vi "Save As CSV.vi"(8 "error in (no error)":errorcluster caption="错误输入（无错误）", 10 "dup path":path, 11 "从板个数":i32) -> (0 "error out":errorcluster caption="错误输出")   [LabVIEW 2013]
uses:
  <vilib>/Utility/file.llb/Write To Spreadsheet File (string).vi
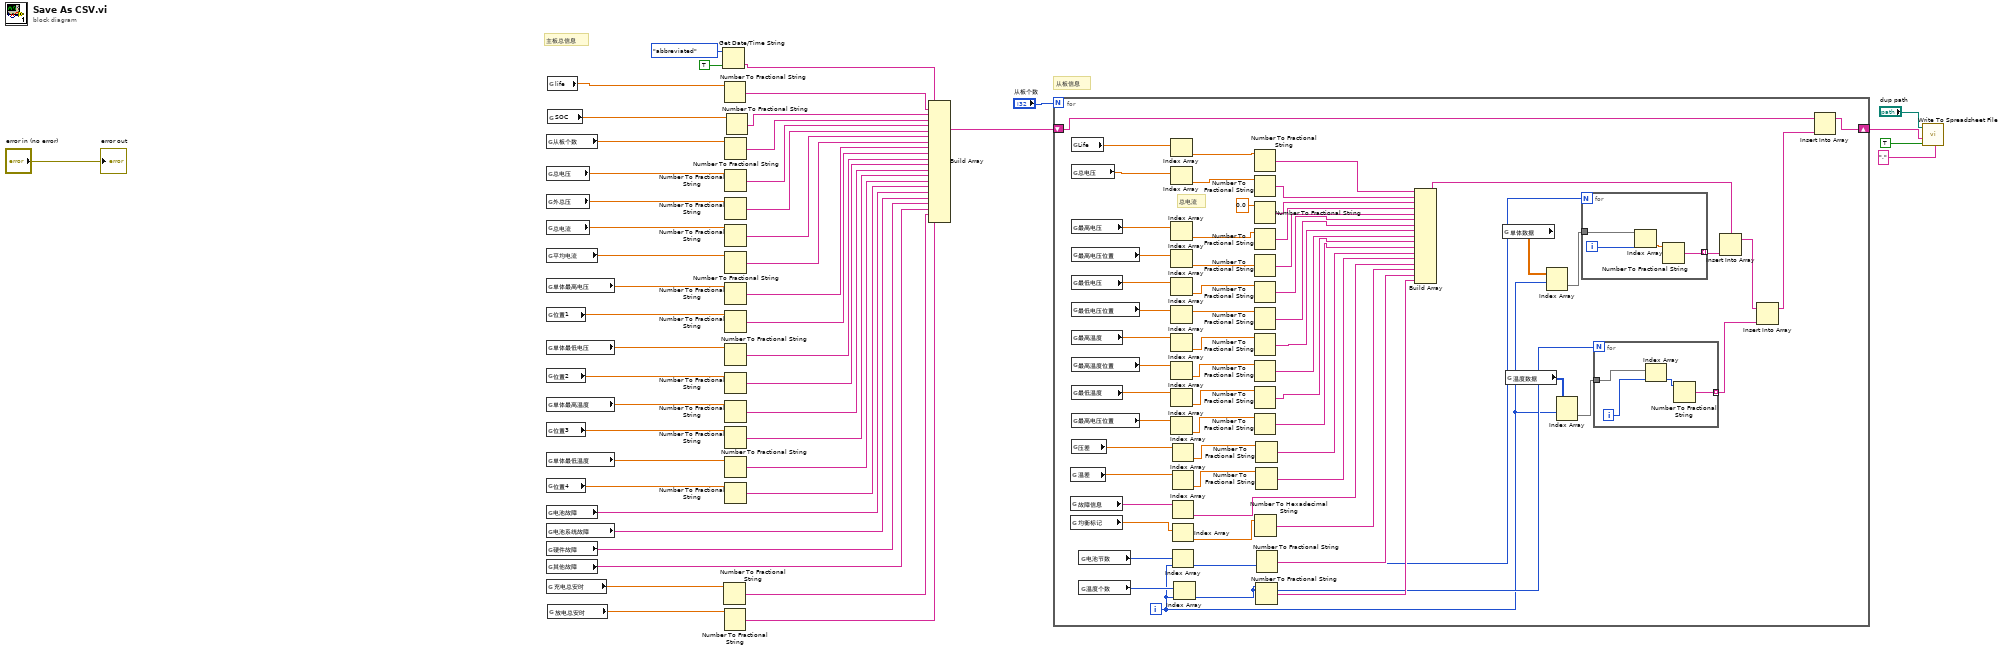
[diagram p0: block diagram]
diagram:
  # "从板信息"
  # "主板总信息"
  n1 = global read "电池信息全局变量.vi" "从板个数"() -> (w20:dbl)
  n2 = global read "EV05全局变量1.vi" "总电压"() -> (w27:dbl)
  n3 = global read "电池信息全局变量.vi" "外总压"() -> (w25:dbl)
  n4 = global read "EV05全局变量1.vi" "总电流"() -> (w26:dbl)
  n5 = global read "电池信息全局变量.vi" "平均电流"() -> (w24:dbl)
  n6 = global read "EV05全局变量1.vi" "单体最高电压"() -> (w17:dbl)
  n7 = global read "EV05全局变量1.vi" "位置1"() -> (w16:dbl)
  n8 = global read "EV05全局变量1.vi" "单体最低电压"() -> (w15:dbl)
  n9 = global read "EV05全局变量1.vi" "位置2"() -> (w14:dbl)
  n10 = global read "EV05全局变量1.vi" "单体最高温度"() -> (w13:dbl)
  n11 = global read "EV05全局变量1.vi" "位置3"() -> (w12:dbl)
  n12 = global read "EV05全局变量1.vi" "单体最低温度"() -> (w11:dbl)
  n13 = global read "EV05全局变量1.vi" "位置4"() -> (w10:dbl)
  n14 = global read "EV05全局变量1.vi" "电池故障"() -> (w9:string)
  n15 = global read "EV05全局变量1.vi" "电池系统故障"() -> (w8:string)
  n16 = global read "EV05全局变量1.vi" "硬件故障"() -> (w7:string)
  n17 = global read "EV05全局变量1.vi" "其他故障"() -> (w6:string)
  n18 = global read "电池信息全局变量.vi" "充电总安时"() -> (w4:dbl)
  n19 = global read "EV05全局变量1.vi" "life"() -> (w19:dbl)
  n20 = global read "EV05全局变量1.vi" "SOC"() -> (w18:dbl)
  n21 = global read "电池信息全局变量.vi" "放电总安时"() -> (w5:dbl)
  n22 = Get Date/Time String(date format (0)=enum16{"short", "long", "abbreviated"}."abbreviated" ("日期格式(0)"), want seconds? (F)=TRUE ("需要秒？(F)")) -> (time string=w46:string)  [unwired: 1 in, 1 out]
  n23 = Number To Fractional String(number=w4) -> (F-format string=w29:string)  [unwired: 3 in]
  n24 = Number To Fractional String(number=w19) -> (F-format string=w3:string)  [unwired: 3 in]
  n25 = Number To Fractional String(number=w5) -> (F-format string=w28:string)  [unwired: 3 in]
  n26 = Number To Fractional String(number=w20) -> (F-format string=w45:string)  [unwired: 3 in]
  n27 = Number To Fractional String(number=w27) -> (F-format string=w44:string)  [unwired: 3 in]
  n28 = Number To Fractional String(number=w25) -> (F-format string=w23:string)  [unwired: 3 in]
  n29 = Number To Fractional String(number=w26) -> (F-format string=w43:string)  [unwired: 3 in]
  n30 = Number To Fractional String(number=w24) -> (F-format string=w22:string)  [unwired: 3 in]
  n31 = Number To Fractional String(number=w17) -> (F-format string=w41:string)  [unwired: 3 in]
  n32 = Number To Fractional String(number=w16) -> (F-format string=w40:string)  [unwired: 3 in]
  n33 = Number To Fractional String(number=w15) -> (F-format string=w39:string)  [unwired: 3 in]
  n34 = Number To Fractional String(number=w14) -> (F-format string=w38:string)  [unwired: 3 in]
  n35 = Number To Fractional String(number=w13) -> (F-format string=w33:string)  [unwired: 3 in]
  n36 = Number To Fractional String(number=w12) -> (F-format string=w32:string)  [unwired: 3 in]
  n37 = Number To Fractional String(number=w11) -> (F-format string=w31:string)  [unwired: 3 in]
  n38 = Number To Fractional String(number=w10) -> (F-format string=w30:string)  [unwired: 3 in]
  n39 = Number To Fractional String(number=w18) -> (F-format string=w2:string)  [unwired: 3 in]
  n40 = Build Array(w46, w3, w2, w45, w44, w23, w43, w22, w41, w40, w39, w38, w33, w32, w31, w30, w9, w8, w7, w6, w29, w28) -> (w21:string[])
  n41 = for {
    N: "从板个数" -> [_]
    shift-right: [w93] -> w37
    shift-left: w21 -> [w92]
    i -> [w49]
    # "总电流"
    n42 = global read "从板全局变量.vi" "温差"() -> (w62:dbl[])
    n43 = global read "从板全局变量.vi" "故障信息"() -> (w59:string[])
    n44 = global read "从板全局变量.vi" "均衡标记"() -> (w56:dbl[])
    n45 = global read "从板全局变量.vi" "Life"() -> (w85:dbl[])
    n46 = global read "从板全局变量.vi" "总电压"() -> (w83:dbl[])
    n47 = global read "从板全局变量.vi" "最高电压"() -> (w79:dbl[])
    n48 = global read "从板全局变量.vi" "最高电压位置"() -> (w80:dbl[])
    n49 = global read "从板全局变量.vi" "最低电压"() -> (w81:dbl[])
    n50 = global read "从板全局变量.vi" "最低电压位置"() -> (w78:dbl[])
    n51 = global read "从板全局变量.vi" "最高温度"() -> (w77:dbl[])
    n52 = global read "从板全局变量.vi" "最高温度位置"() -> (w76:dbl[])
    n53 = global read "从板全局变量.vi" "最低温度"() -> (w74:dbl[])
    n54 = global read "从板全局变量.vi" "最高电压位置"() -> (w75:dbl[])
    n55 = global read "从板全局变量.vi" "压差"() -> (w63:dbl[])
    n56 = global read "从板全局变量.vi" "电池节数"() -> (w88:u8[])
    n57 = global read "从板全局变量.vi" "温度个数"() -> (w89:u8[])
    n58 = Index Array(array=w85) -> (element=w84:dbl)  [unwired: 1 in]
    n59 = Index Array(array=w83) -> (element=w82:dbl)  [unwired: 1 in]
    n60 = Index Array(array=w79) -> (element=w73:dbl)  [unwired: 1 in]
    n61 = Index Array(array=w80) -> (element=w72:dbl)  [unwired: 1 in]
    n62 = Index Array(array=w81) -> (element=w71:dbl)  [unwired: 1 in]
    n63 = Index Array(array=w78) -> (element=w70:dbl)  [unwired: 1 in]
    n64 = Index Array(array=w77) -> (element=w69:dbl)  [unwired: 1 in]
    n65 = Index Array(array=w76) -> (element=w68:dbl)  [unwired: 1 in]
    n66 = Index Array(array=w74) -> (element=w67:dbl)  [unwired: 1 in]
    n67 = Index Array(array=w75) -> (element=w66:dbl)  [unwired: 1 in]
    n68 = Index Array(array=w63) -> (element=w64:dbl)  [unwired: 1 in]
    n69 = Index Array(array=w62) -> (element=w65:dbl)  [unwired: 1 in]
    n70 = Index Array(array=w59) -> (element=w58:string)  [unwired: 1 in]
    n71 = Index Array(array=w56) -> (element=w55:dbl)  [unwired: 1 in]
    n72 = Index Array(array=w88, index=w49) -> (element=w87:u8)
    n73 = Index Array(array=w89, index=w49) -> (element=w86:u8)
    n74 = Number To Fractional String(number=w84) -> (F-format string=w90:string)  [unwired: 3 in]
    n75 = Number To Fractional String(number=w82) -> (F-format string=w109:string)  [unwired: 3 in]
    n76 = Number To Fractional String(number=0.0 ("数字")) -> (F-format string=w108:string)  [unwired: 3 in]
    n77 = Number To Fractional String(number=w73) -> (F-format string=w107:string)  [unwired: 3 in]
    n78 = Number To Fractional String(number=w72) -> (F-format string=w106:string)  [unwired: 3 in]
    n79 = Number To Fractional String(number=w71) -> (F-format string=w105:string)  [unwired: 3 in]
    n80 = Number To Fractional String(number=w70) -> (F-format string=w104:string)  [unwired: 3 in]
    n81 = Number To Fractional String(number=w69) -> (F-format string=w103:string)  [unwired: 3 in]
    n82 = Number To Fractional String(number=w68) -> (F-format string=w102:string)  [unwired: 3 in]
    n83 = Number To Fractional String(number=w67) -> (F-format string=w101:string)  [unwired: 3 in]
    n84 = Number To Fractional String(number=w66) -> (F-format string=w100:string)  [unwired: 3 in]
    n85 = Number To Hexadecimal String(2:w55) -> (0:w57:string)  [unwired: 1 in]
    n86 = Number To Fractional String(number=w64) -> (F-format string=w61:string)  [unwired: 3 in]
    n87 = Number To Fractional String(number=w65) -> (F-format string=w60:string)  [unwired: 3 in]
    n88 = Number To Fractional String(number=w86) -> (F-format string=w98:string)  [unwired: 3 in]
    n89 = Number To Fractional String(number=w87) -> (F-format string=w99:string)  [unwired: 3 in]
    n90 = Build Array(w90, w109, w108, w107, w106, w105, w104, w103, w102, w101, w100, w61, w60, w58, w57, w99, w98) -> (w96:string[])
    n91 = global read "单体信息全局.vi" "单体数据"() -> (w53:dbl[][])
    n92 = global read "单体信息全局.vi" "温度数据"() -> (w51:u8[][])
    n93 = Index Array(array=w53, index (row)=w49) -> (element=w52:dbl[])  [unwired: 1 in]
    n94 = Index Array(array=w51, index (row)=w49) -> (element=w50:u8[])  [unwired: 1 in]
    n95 = for {
      N: w87 -> [_]
      tunnel: [w117] -> w97 mode=indexing
      tunnel: w52 -> [w116]
      i -> [w114]
      n96 = Index Array(array=w116, index=w114) -> (element=w115:dbl)
      n97 = Number To Fractional String(number=w115) -> (F-format string=w117:string)  [unwired: 3 in]
    }
    n98 = for {
      N: w86 -> [_]
      tunnel: [w113] -> w95 mode=indexing
      tunnel: w50 -> [w111]
      i -> [w110]
      n99 = Index Array(array=w111, index=w110) -> (element=w112:u8)
      n100 = Number To Fractional String(number=w112) -> (F-format string=w113:string)  [unwired: 3 in]
    }
    n101 = Insert Into Array(array=w96, new element=w97) -> (w94:string[])  [unwired: 1 in]
    n102 = Insert Into Array(array=w94, new element=w95) -> (w91:string[])  [unwired: 1 in]
    n103 = Insert Into Array(array=w92, new element=w91) -> (w93:string[])  [unwired: 1 in]
  }
  n104 = call-poly <vilib>:"Write To Spreadsheet File.vi"("delimiter (\\t)"="," ("delimiter (\\t)"), "append to file? (new file:F)"=TRUE, "1D data"=w37, "file path (dialog if empty)"="dup path") -> ()  [unwired: 4 in, 1 out]
  "error out" <- "error in (no error)"
